vi "LWXPS_Example_zone.vi"() -> ()   [LabVIEW 2013]
panel:
  out "Hysteresis in µm":dbl
  out "Radius in µm":dbl
  out "Y center in µm":dbl
  out "X center in µm":dbl
  in  "Hysteresis":dbl
  in  "Radius":dbl
  in  "Y center":dbl
  in  "X center":dbl
  out "XPS Error String":string
  out "Returned error code":i32
  out "Error out":errorcluster caption="error out"
  out "Error code":i32
  in  "Instrument Key IN":string
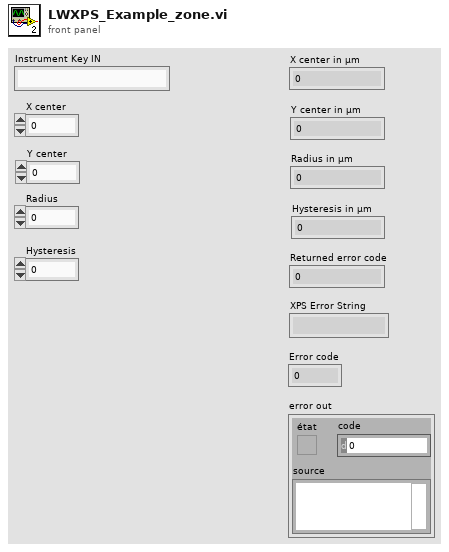
[diagram p1: front panel]
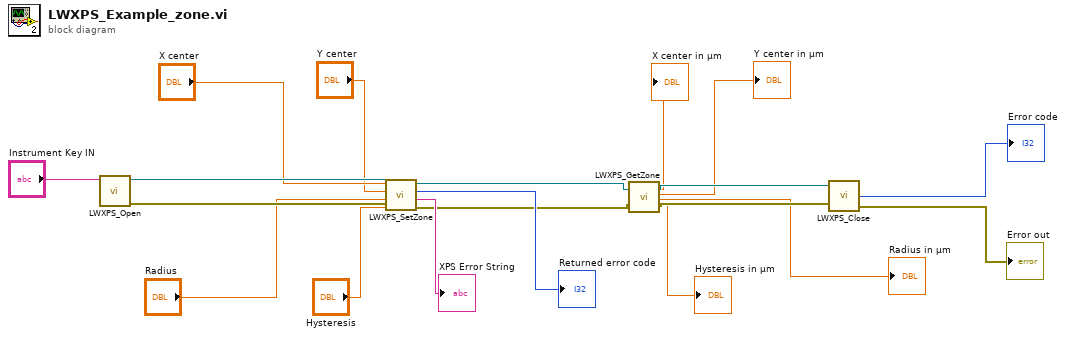
[diagram p0: block diagram]
diagram:
  n1 = call "LWXPS_Open.vi"("Instrument Key IN"="Instrument Key IN") -> ("error out"=w17:errorcluster, "CommandInterfaceXPS.XPS"=w19:refnum<k24>)  [unwired: 3 in, 2 out]
  n2 = call "LWXPS_SetZone.vi"("LabVIEW error IN"=w17, "XPS Reference IN"=w19, "Hysteresis"="Hysteresis", "Radius"="Radius", "Y center"="Y center", "X center"="X center") -> ("LabVIEW error OUT"=w7:errorcluster, "XPS Error String"=→"XPS Error String":string, "Returned error code"=→"Returned error code":i32, "CommandInterfaceXPS.XPS"=w8:refnum<k24>)  [unwired: 1 in]
  n3 = call "LWXPS_GetZone.vi"("XPS Reference IN"=w8, "LabVIEW error IN"=w7) -> ("CommandInterfaceXPS.XPS"=w6:refnum<k24>, "LabVIEW error OUT"=w5:errorcluster, "X center in µm"=→"X center in µm":dbl, "Y center in µm"=→"Y center in µm":dbl, "Radius in µm"=→"Radius in µm":dbl, "Hysteresis in µm"=→"Hysteresis in µm":dbl)  [unwired: 10 in, 2 out]
  n4 = call "LWXPS_Close.vi"("error in (no error)"=w5, "XPS Reference"=w6) -> ("Error out"=→"Error out":errorcluster, "Error code"=→"Error code":i32)  [unwired: 2 in]
